vi "tsc--Show Color Picker.vi"(8 "error in":errorcluster, 10 "Color start":u32(colorbox), 11 "VI Refnum":refnum<vi>) -> (0 "error out":errorcluster, 1 "OK?":bool, 2 "Color out":u32(colorbox))   [LabVIEW 2021]
doc: "Show the color picker tool to select the new image color.\n\n<b>Code Developed By:</b>\nTechnology Service Corporation\n1983 S Liberty Drive\nBloomington, IN 47403\nPhone: 812 558-7100\nwww.tsc.com/atcs\n\nDeveloper:\nDaniel Coons"
uses:
  System.Windows.Forms
  System.Drawing
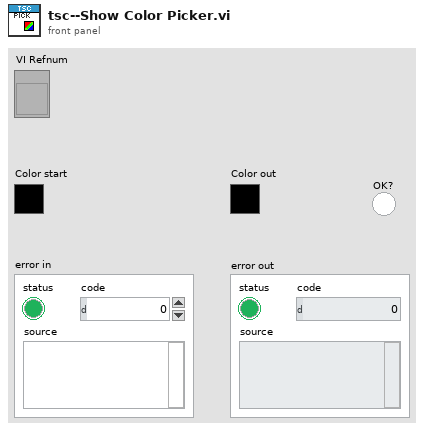
[diagram p1: front panel]
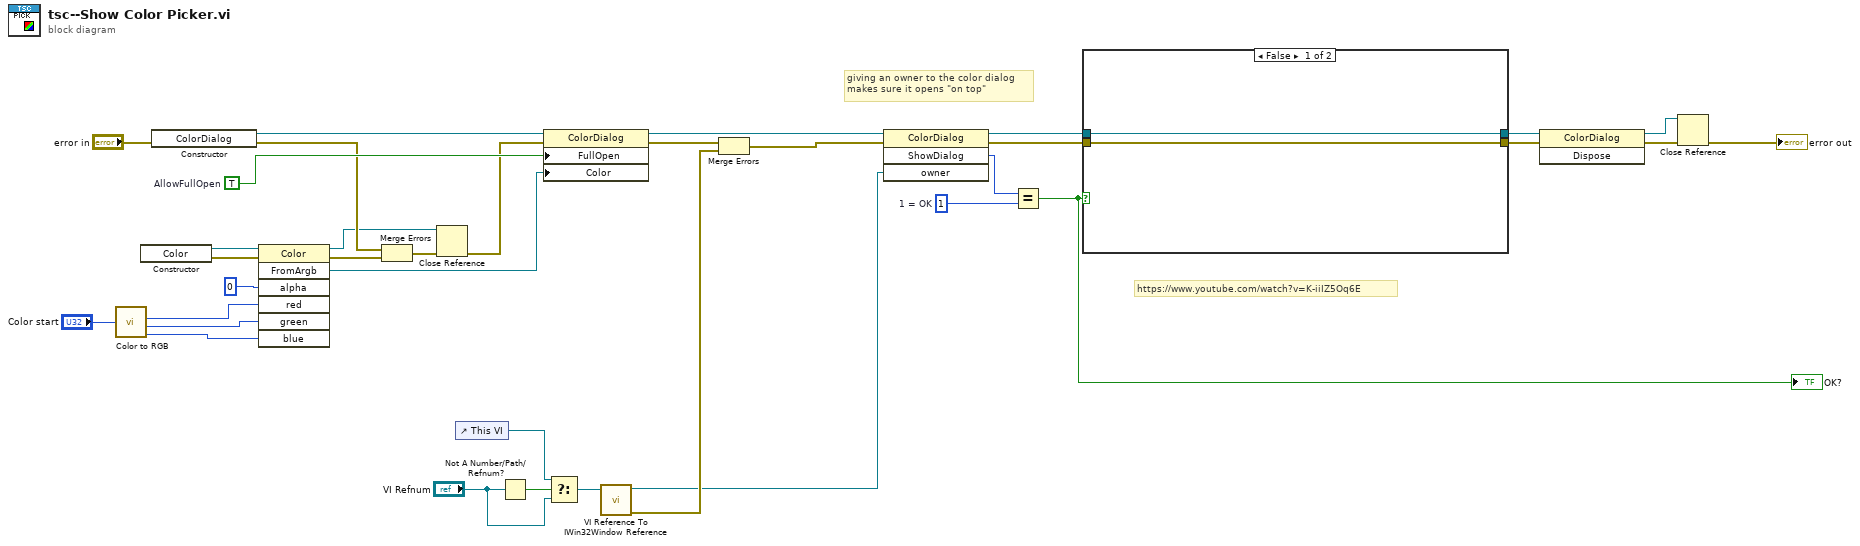
[diagram p0: block diagram]
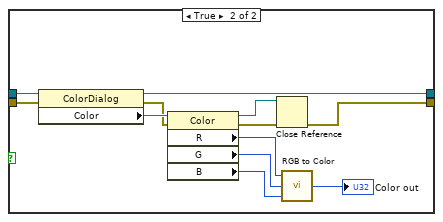
[diagram p2: hidden frame]
diagram:
  w29 = TRUE  # AllowFullOpen
  w34 = 1  # 1 = OK
  # "giving an owner to the color dialog\nmakes sure it opens \"on top\""
  # "https://www.youtube.com/watch?v=K-iiIZ5Oq6E"
  n1 = call <vilib>:"Color to RGB.vi"("Color"="Color start") -> ("R"=w19:u8, "G"=w18:u8, "B"=w17:u8)  [unwired: 1 out]
  n2 = constructor class="Color"() -> (reference out=w22:refnum<k24>, error out=w21:errorcluster)  [unwired: 3 in, 1 out]
  n3 = constructor class="ColorDialog"(error in="error in") -> (reference out=w31:refnum<k24>, error out=w13:errorcluster)  [unwired: 2 in, 1 out]
  n4 = invoke class="Color" method="FromArgb"(reference=w22, error in=w21, "alpha"=0, "red"=w19, "green"=w18, "blue"=w17) -> (reference out=w10:refnum<k24>, error out=w14:errorcluster, "FromArgb"=w16:refnum<k24>)  [unwired: 1 in, 4 out]
  n5 = Merge Errors(w13, w14) -> (w12:errorcluster)
  n6 = Close Reference(reference=w10, error in (no error)=w12) -> (error out=w11:errorcluster)
  n7 = control-ref of="This VI"() -> (w5:refnum<vi>)
  n8 = Not A Number/Path/Refnum?(number/path/refnum="VI Refnum") -> (NaN/Path/Refnum?=w6:bool)
  n9 = property class="ColorDialog"(reference=w31, error in=w11, "FullOpen"=w29, "Color"=w16) -> (reference out=w30:refnum<k24>, error out=w32:errorcluster)
  n10 = Select(t=w5, s=w6, f="VI Refnum") -> (s? t:f=w3:refnum<vi>)
  n11 = call "VI Reference To IWin32Window Reference.vi"("VI Reference"=w3) -> ("error out"=w2:errorcluster, "System.Windows.Forms.IWin32Window"=w1:refnum<k24>)  [unwired: 9 in]
  n12 = Merge Errors(w32, w2) -> (w7:errorcluster)
  n13 = invoke class="ColorDialog" method="ShowDialog"(reference=w30, error in=w7, "owner"=w1) -> (reference out=w8:refnum<k24>, error out=w9:errorcluster, "ShowDialog"=w35:i32)  [unwired: 1 in, 1 out]
  n14 = Equal?(x=w35, y=w34) -> (x = y?=w33:bool)
  "OK?" <- w33
  n15 = case shown="False" w33 {
    tunnel: w8 -> [w37 w49]
    tunnel: [w37 w40] -> w28
    tunnel: [w36 w39] -> w27
    tunnel: w9 -> [w36 w38]
    frame False {
    }
    frame True {
      n16 = property class="ColorDialog"(reference=w49, error in=w38) -> (reference out=w40:refnum<k24>, error out=w47:errorcluster, "Color"=w48:refnum<k24>)
      n17 = property class="Color"(reference=w48, error in=w47) -> (reference out=w45:refnum<k24>, error out=w46:errorcluster, "R"=w42:u8, "G"=w43:u8, "B"=w44:u8)
      n18 = Close Reference(reference=w45, error in (no error)=w46) -> (error out=w39:errorcluster)
      n19 = call <vilib>:"RGB to Color.vi"("B"=w44, "G"=w43, "R"=w42) -> ("Color"=→"Color out":u32)
    }
  }
  n20 = invoke class="ColorDialog" method="Dispose"(reference=w28, error in=w27) -> (reference out=w25:refnum<k24>, error out=w26:errorcluster)  [unwired: 1 in, 1 out]
  n21 = Close Reference(reference=w25, error in (no error)=w26) -> (error out=→"error out":errorcluster)
